vi "Commit NVMEM.vi"   [LabVIEW 2020, in "SLSC.lvlib"]
doc: "Commits pending changes to hardware for non-volatile memory. If you set the same address multiple times between commits, only the last value will be committed."
uses:
  <vilib>/SLSC/SLSC.lvlib
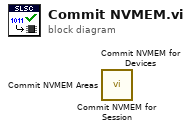
[diagram p0: block diagram]
diagram:
  n1 = call <vilib>:"Commit NVMEM for Session.vi"() -> ()  [unwired: 14 in, 2 out]
  n2 = call <vilib>:"Commit NVMEM for Devices.vi"() -> ()  [unwired: 14 in, 2 out]
  n3 = call <vilib>:"Commit NVMEM Areas.vi"() -> ()  [unwired: 14 in, 2 out]
